vi "精确匹配单词.vi"() -> ()   [LabVIEW 2012]
uses:
  <vilib>/regexp/Match Regular Expression.xnode
panel:
  out "匹配后偏移量":i32=600
  out "匹配之后":string=" data associated with the statechart. \n\n"
  out "所有匹配":string="state"
  out "匹配之前":string="When you build a statechart, you define unique states in which the statechart can be. You also define transitions between these states, when the statechart can take these transitions, and what actions these transitions can take. You then define triggers that cause the statechart to begin evaluating a certain transition. For example, consider a statechart that you use to control a chemical process. You can specify that the statechart moves from State 1 to State 2 after receiving the Valve Open trigger. States and transitions also have associated actions, which you use to modify output and "
  in  "正则表达式":string="\\bstate\\b"
  in  "字符串":string="When you build a statechart, you define unique states in which the statechart can be. You also define transitions between these states, when the statechart can take these transitions, and what actions these transitions can take. You then define triggers that cause the statechart to begin evaluating a certain transition. For example, consider a statechart that you use to control a chemical process. You can specify that the statechart moves from State 1 to State 2 after receiving the Valve Open trigger. States and transitions also have associated actions, which you use to modify output and state data associated with the statechart. \n\n"
  # "\\b代表单词的开头或结尾，通常由空格、标点符号或者换行来分隔。"
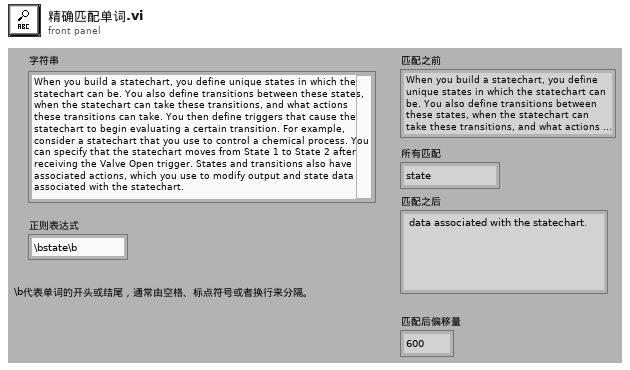
[diagram p1: front panel]
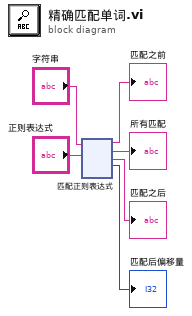
[diagram p0: block diagram]
diagram:
  n1 = xnode "匹配正则表达式"("输入字符串"="字符串", "正则表达式"="正则表达式") -> ("匹配之前"=→"匹配之前":string, "所有匹配"=→"所有匹配":string, "匹配之后"=→"匹配之后":string, "匹配后偏移量"=→"匹配后偏移量":i32)  [unwired: 4 in, 1 out]
